vi "Preview.vi"(8 "error in (no error)":errorcluster, 10 "Project":refnum<vi>, 11 "IB_Tree_Item_Proj_Folder_Sync in":refnum<class "IB_Tree_Item_Proj_Folder_Sync.lvclass">) -> (0 "error out":errorcluster, 2 "first preview?":bool, 3 "IB_Tree_Item_Proj_Folder_Sync out":refnum<class "IB_Tree_Item_Proj_Folder_Sync.lvclass">)   [LabVIEW 2020, in "IB_Tree_Item_Proj_Folder_Sync.lvclass"]
uses:
  <vilib>/AppBuilder/IB_Classes/Tree_Item_Proj_Folder_Sync/IB_Tree_Item_Proj_Folder_Sync.lvclass
  <vilib>/AppBuilder/IB_Classes/Tree_Item_Proj_Folder_Sync/IB_Tree_Item_Proj_Folder_Sync.lvclass/IB_Tree_Item_Proj_Folder_Sync.ctl
  <vilib>/AppBuilder/IB_Classes/Tree_Item_Proj/IB_Tree_Item_Proj.lvclass
  <vilib>/AppBuilder/IB_Classes/Tree_Item_Proj_Container/IB_Tree_Item_Proj_Container.lvclass
  <vilib>/AppBuilder/IB_Classes/Tree_Item_Proj_Contained_File/IB_Tree_Item_Proj_Contained_File.lvclass
  <vilib>/AppBuilder/IB_Classes/Tree_Item_Virtual_Folder/IB_Tree_Item_Virtual_Folder.lvclass
  <vilib>/AppBuilder/IB_Classes/Tree_Item/IB_Tree_Item.lvclass
  <vilib>/AppBuilder/IB_Classes/Tree_Item_Proj_Folder/IB_Tree_Item_Proj_Folder.lvclass
  e:/builds/penguin/labview/branches/2020/dev/dist/vi.lib/AppBuilder/IB_Classes/Tree_Item_Proj_Folder/IB_Tree_Item_Proj_Folder.lvclass
  e:/builds/penguin/labview/branches/2020/dev/dist/vi.lib/AppBuilder/IB_Classes/Tree_Item_Proj_Container/IB_Tree_Item_Proj_Container.lvclass
  e:/builds/penguin/labview/branches/2020/dev/dist/vi.lib/AppBuilder/IB_Classes/Tree_Item_Proj/IB_Tree_Item_Proj.lvclass
  e:/builds/penguin/labview/branches/2020/dev/dist/vi.lib/AppBuilder/IB_Classes/Tree_Item/IB_Tree_Item.lvclass
  e:/builds/penguin/labview/branches/2020/dev/dist/vi.lib/AppBuilder/IB_Classes/Tree_Item_Proj_Folder_Sync/IB_Tree_Item_Proj_Folder_Sync.lvclass
  e:/builds/penguin/labview/branches/2020/dev/dist/vi.lib/AppBuilder/IB_Classes/Tree_Item_Proj_File/IB_Tree_Item_Proj_File.lvclass
  e:/builds/penguin/labview/branches/2020/dev/dist/vi.lib/AppBuilder/IB_Classes/Tree_Item_Proj_Contained_File/IB_Tree_Item_Proj_Contained_File.lvclass
  e:/builds/penguin/labview/branches/2020/dev/dist/vi.lib/AppBuilder/IB_Classes/Tree_Item_Virtual_Folder/IB_Tree_Item_Virtual_Folder.lvclass
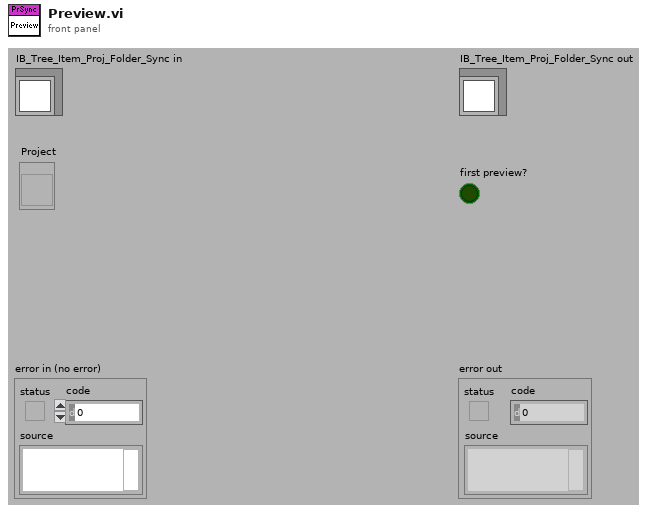
[diagram p1: front panel]
types:
  T1 = typedef "IB_Tree_Item_Proj.ctl" = cluster{"itemID":string, "path":path}
  T2 = typedef "IB_Tree_Item.ctl" = cluster{"symbol index":i32, "child tag":string, "parentTag":string, "left cell name":string}
  T3 = typedef "IB_Tree_Item_Proj_Contained_File.ctl" = cluster{"virt folders":refnum<class "IB_Tree_Item_Virtual_Folder.lvclass">[]}
  T4 = typedef "IB_Tree_Item_Proj_Container.ctl" = cluster{"ctr files":refnum<class "IB_Tree_Item_Proj_Contained_File.lvclass">[], "previewed?":bool, "expanded?":bool, "preview error?":bool}
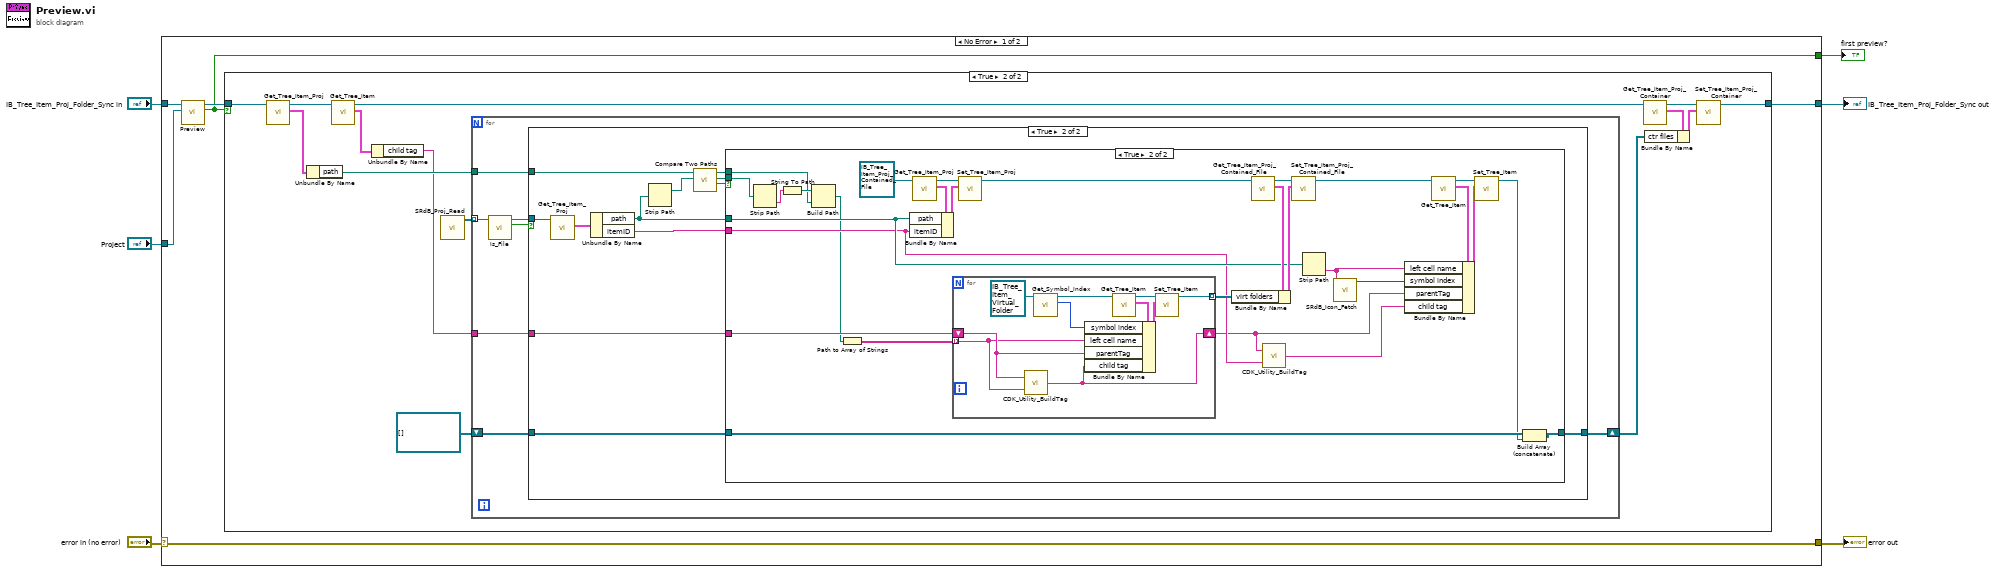
[diagram p0: block diagram]
diagram:
  n1 = case shown="No Error" "error in (no error)" {
    selector: "error in (no error)" -> [w12 w89]
    tunnel: [w12 w89] -> w5
    tunnel: [w11 w88] -> w3
    tunnel: "IB_Tree_Item_Proj_Folder_Sync in" -> [w9 w88]
    tunnel: "Project" -> [w8 _]
    tunnel: [w7 _] -> w1
    frame No Error {
      n2 = call-parent "Preview.vi"("Project"=w8, "IB_Tree_Item_Proj_Container in"=w9) -> ("first preview?"=w7:bool, "IB_Tree_Item_Proj_Container out"=w10:refnum<class "IB_Tree_Item_Proj_Folder_Sync.lvclass">)  [unwired: 1 in, 7 out]
      n3 = case shown="True" w7 {
        tunnel: [w13 w27] -> w11
        tunnel: w10 -> [w13 w26]
        frame False {
        }
        frame True {
          n4 = call <vilib>:"Get_Tree_Item_Proj.vi"("IB_TreeProjectItem in"=w26) -> ("data"=w24:T1, "IB_TreeProjectItem out"=w17:refnum<class "IB_Tree_Item_Proj_Folder_Sync.lvclass">)  [unwired: 1 in, 8 out]
          n5 = Unbundle By Name(w24) -> ("path"=w23:path)
          n6 = call <vilib>:"Get_Tree_Item.vi"("IB_TreeItem in"=w17) -> ("data"=w15:T2, "IB_TreeItem out"=w16:refnum<class "IB_Tree_Item_Proj_Folder_Sync.lvclass">)  [unwired: 1 in, 8 out]
          n7 = Unbundle By Name(w15) -> ("child tag"=w14:string)
          n8 = call <resource>:"SRdB_Proj_Read.vi"() -> ("Proj Items"=w25:refnum<class "IB_Tree_Item_Proj.lvclass">[])  [unwired: 1 in, 10 out]
          n9 = for {
            tunnel: w25 -> [w31] mode=indexing
            tunnel: w23 -> [w34]
            shift-right: [w32] -> w18
            shift-left: refnum<class "IB_Tree_Item_Proj_Contained_File.lvclass">[] [] ("ctr files") -> [w33]
            tunnel: w14 -> [w28]
            n10 = call-dynamic "Is_File.vi"("IB_Tree_Item_Proj in"=w31) -> ("file?"=w29:bool, "IB_Tree_Item_Proj out"=w30:refnum<class "IB_Tree_Item_Proj.lvclass">)  [unwired: 1 in, 8 out]
            n11 = case shown="True" w29 {
              tunnel: w34 -> [_ w37]
              tunnel: w33 -> [w35 w44]
              tunnel: [w35 w43] -> w32
              tunnel: w30 -> [_ w42]
              tunnel: w28 -> [_ w41]
              frame False {
              }
              frame True {
                n12 = call <vilib>:"Get_Tree_Item_Proj.vi"("IB_TreeProjectItem in"=w42) -> ("data"=w47:T1)  [unwired: 1 in, 9 out]
                n13 = Unbundle By Name(w47) -> ("path"=w39:path, "itemID"=w40:string)
                n14 = Strip Path(path=w39) -> (stripped path=w38:path)  [unwired: 1 out]
                n15 = call <vilib>:"Compare Two Paths.vi"("Path 2"=w38, "Path 1"=w37) -> ("Path 2 Relative to Path 1?"=w45:bool, "Common Path"=w36:path, "Relative Path from 1 to 2"=w46:path)  [unwired: 3 in, 4 out]
                n16 = case shown="True" w45 {
                  tunnel: w46 -> [_ w50]
                  tunnel: w44 -> [w48 w72]
                  tunnel: [w48 w71] -> w43
                  tunnel: w41 -> [_ w70]
                  tunnel: w39 -> [_ w57]
                  tunnel: w40 -> [_ w56]
                  tunnel: w36 -> [_ w53]
                  frame False {
                  }
                  frame True {
                    n17 = Strip Path(path=w53) -> (name=w52:string)  [unwired: 1 out]
                    n18 = String To Path(string=w52) -> (path=w51:path)
                    n19 = Build Path(base path=w51, name or relative path=w50) -> (appended path=w49:path)
                    n20 = Path to Array of Strings(0:w49) -> (2:w73:string[])  [unwired: 1 out]
                    n21 = call <vilib>:"Get_Tree_Item_Proj.vi"("IB_TreeProjectItem in"=refnum<class "IB_Tree_Item_Proj_Contained_File.lvclass"> refnum ("IB_Tree_Item_Proj_Contained_File.lvclass")) -> ("data"=w66:T1, "IB_TreeProjectItem out"=w67:refnum<class "IB_Tree_Item_Proj_Contained_File.lvclass">)  [unwired: 1 in, 8 out]
                    n22 = Bundle By Name(cluster=w66, "path"=w57, "itemID"=w56) -> (w68:T1)
                    n23 = for {
                      tunnel: [w87] -> w74 mode=indexing
                      tunnel: w73 -> [w84] mode=indexing
                      shift-right: [w86] -> w55
                      shift-left: w70 -> [w85]
                      n24 = call <resource>:"CDK_Utility_BuildTag.vi"("name or relative path"=w84, "BasePath"=w85) -> ("appended path"=w86:string)
                      n25 = call-dynamic "Get_Symbol_Index.vi"("IB_TreeVirtFolderItem in"=refnum<class "IB_Tree_Item_Virtual_Folder.lvclass"> refnum ("IB_Tree_Item_Virtual_Folder.lvclass")) -> ("symbol index"=w78:i32, "IB_TreeVirtFolderItem out"=w79:refnum<class "IB_Tree_Item_Virtual_Folder.lvclass">)  [unwired: 1 in, 8 out]
                      n26 = call <vilib>:"Get_Tree_Item.vi"("IB_TreeItem in"=w79) -> ("data"=w82:T2, "IB_TreeItem out"=w83:refnum<class "IB_Tree_Item_Virtual_Folder.lvclass">)  [unwired: 1 in, 8 out]
                      n27 = Bundle By Name(cluster=w82, "symbol index"=w78, "left cell name"=w84, "parentTag"=w85, "child tag"=w86) -> (w81:T2)
                      n28 = call <vilib>:"Set_Tree_Item.vi"("data"=w81, "IB_TreeItem in"=w83) -> ("IB_TreeItem out"=w87:refnum<class "IB_Tree_Item_Virtual_Folder.lvclass">)  [unwired: 1 in, 8 out]
                    }
                    n29 = call <vilib>:"Set_Tree_Item_Proj.vi"("data"=w68, "IB_TreeProjectItem in"=w67) -> ("IB_TreeProjectItem out"=w65:refnum<class "IB_Tree_Item_Proj_Contained_File.lvclass">)  [unwired: 1 in, 8 out]
                    n30 = call <vilib>:"Get_Tree_Item_Proj_Contained_File.vi"("IB_Tree_Item_Proj_Contained_File in"=w65) -> ("data"=w76:T3, "IB_Tree_Item_Proj_Contained_File out"=w77:refnum<class "IB_Tree_Item_Proj_Contained_File.lvclass">)  [unwired: 1 in, 8 out]
                    n31 = Bundle By Name(cluster=w76, "virt folders"=w74) -> (w75:T3)
                    n32 = call <resource>:"CDK_Utility_BuildTag.vi"("name or relative path"=w56, "BasePath"=w55) -> ("appended path"=w54:string)
                    n33 = call <vilib>:"Set_Tree_Item_Proj_Contained_File.vi"("data"=w75, "IB_Tree_Item_Proj_Contained_File in"=w77) -> ("IB_Tree_Item_Proj_Contained_File out"=w59:refnum<class "IB_Tree_Item_Proj_Contained_File.lvclass">)  [unwired: 1 in, 8 out]
                    n34 = Strip Path(path=w57) -> (name=w63:string)  [unwired: 1 out]
                    n35 = call <resource>:"SRdB_Icon_Fetch.vi"("filename"=w63) -> ("symbol index"=w64:i32)  [unwired: 1 in, 9 out]
                    n36 = call <vilib>:"Get_Tree_Item.vi"("IB_TreeItem in"=w59) -> ("data"=w61:T2, "IB_TreeItem out"=w60:refnum<class "IB_Tree_Item_Proj_Contained_File.lvclass">)  [unwired: 1 in, 8 out]
                    n37 = Bundle By Name(cluster=w61, "left cell name"=w63, "symbol index"=w64, "parentTag"=w55, "child tag"=w54) -> (w62:T2)
                    n38 = call <vilib>:"Set_Tree_Item.vi"("data"=w62, "IB_TreeItem in"=w60) -> ("IB_TreeItem out"=w58:refnum<class "IB_Tree_Item_Proj_Contained_File.lvclass">)  [unwired: 1 in, 8 out]
                    n39 = Build Array (concatenate)(w72, w58) -> (w71:refnum<class "IB_Tree_Item_Proj_Contained_File.lvclass">[])
                  }
                }
              }
            }
          }
          n40 = call <vilib>:"Get_Tree_Item_Proj_Container.vi"("IB_Tree_Item_Proj_Container in"=w16) -> ("data"=w21:T4, "IB_Tree_Item_Proj_Container out"=w22:refnum<class "IB_Tree_Item_Proj_Folder_Sync.lvclass">)  [unwired: 1 in, 8 out]
          n41 = Bundle By Name(cluster=w21, "ctr files"=w18) -> (w20:T4)
          n42 = call <vilib>:"Set_Tree_Item_Proj_Container.vi"("data"=w20, "IB_Tree_Item_Proj_Container in"=w22) -> ("IB_Tree_Item_Proj_Container out"=w27:refnum<class "IB_Tree_Item_Proj_Folder_Sync.lvclass">)  [unwired: 1 in, 8 out]
        }
      }
    }
    frame Error {
    }
  }
  "error out" <- w5
  "IB_Tree_Item_Proj_Folder_Sync out" <- w3
  "first preview?" <- w1
